vi "KE6517_CommandsGlobal.vi"() -> ()   [LabVIEW 2013, in "KE6517.lvclass"]
uses:
  KE6517.lvclass
panel:
  in  "Keithley 6517 GPIB Setup":T1={"GPIB address"="27", "Instrument name"="Keithley 6517", "Instrument type"=0, "Command \"Reset\""="*rst", "Command \"Initialise\""=":Calculate:state 0; :trigger:source imm; :trigger:count inf; :format:data ASCii; :format:elements reading; :source:voltage:range 1000; :sense:func 'curr:dc'; :sense:current:range:auto:llimit 200e-6; :sense:current:range:auto 1; :source:voltage:mconnect 0; :source:current:rlimit:state %d;", "Command \"Arm\""=":system:zcheck 0; :init; :sour:volt:lev:imm:ampl 0; :output:state ON;", "Command \"SetVolts\""=":sour:volt:lev:imm:ampl %3.2f", "Command \"Compliance?\""=":source:current:limit:state?", "Command \"Standby\""=":sour:volt:lev:imm:ampl 0.0; :output:state 0; :system:zcheck 1\n", "Command \"Read Current\""=":sense:data:latest?"} {"Instrument type" items=["Supply", "LCR"]}
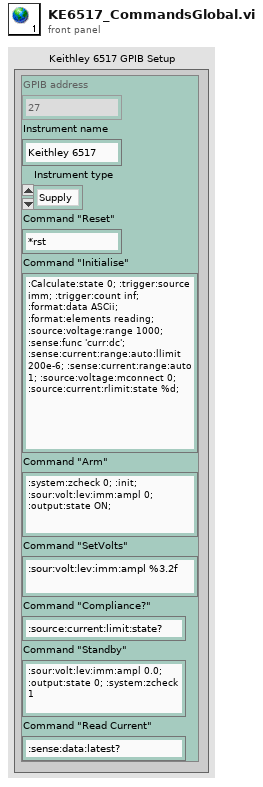
[diagram p1: front panel]
types:
  T1 = cluster{"GPIB address":string, "Instrument name":string, "Instrument type":u16, "Command \"Reset\"":string, "Command \"Initialise\"":string, "Command \"Arm\"":string, "Command \"SetVolts\"":string, "Command \"Compliance?\"":string, "Command \"Standby\"":string, "Command \"Read Current\"":string}
diagram:
